vi "DiffDrivePoseEst_FillStateVector.vi"(9 "RightDist":dbl, 10 "LeftDist":dbl, 11 "InitialPose":T2={"TRANSLATION"={"X"=0.0, "Y"=0.0}, "ROTATION"={"VALUE"=0.0, "COS"=1.0, "SIN"=0.0}} {"ROTATION"."SIN" format="%13.4f"; "ROTATION"."COS" format="%13.4f"; "ROTATION"."VALUE" format="%13.4f"; "TRANSLATION"."Y" format="%14.3f"; "TRANSLATION"."X" format="%14.3f"}) -> (3 "output matrix":T1)   [LabVIEW 2019, in "Trajectory_Library.lvlib"]
doc: "Create a vector with the current robot pose, encoder distances, and gyro\n\nInputs:\n - initialPose -- robot pose\n - LeftDist -- left encoder distance\n - RightDist -- right encoder distance\n\nOutputs:\n - output Matrix -- filled matrix."
uses:
  Trajectory_Library.lvlib
  POSE2D.ctl
  TRANSLATION2D.ctl
  ROTATION2D.ctl
  <vilib>/Analysis/Matrix/Datatypes/RealMatrix.ctl
  MatBuilder_Create.vi
  <vilib>/Analysis/Matrix/NI_Matrix.lvlib
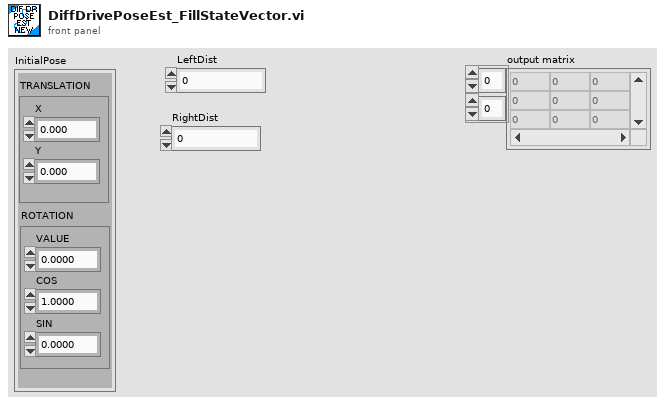
[diagram p1: front panel]
types:
  T1 = typedef "NI_Matrix.lvlib/RealMatrix.ctl" = dbl[][]
  T2 = typedef "Trajectory_Library.lvlib/POSE2D.ctl" = cluster{"TRANSLATION":T3, "ROTATION":T4}
  T3 = typedef "Trajectory_Library.lvlib/TRANSLATION2D.ctl" = cluster{"X":dbl, "Y":dbl}
  T4 = typedef "Trajectory_Library.lvlib/ROTATION2D.ctl" = cluster{"VALUE":dbl, "COS":dbl, "SIN":dbl}
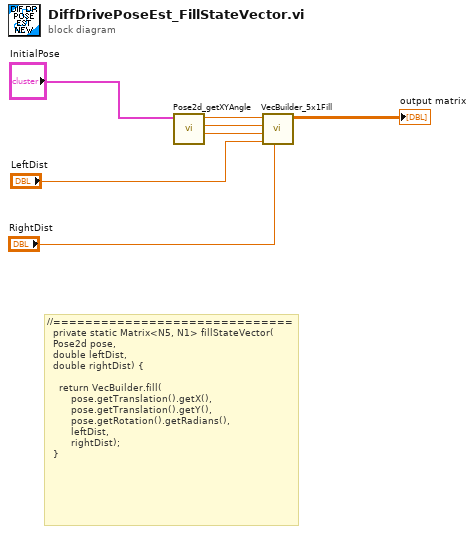
[diagram p0: block diagram]
diagram:
  # "//==============================\n  private static Matrix<N5, N1> fillStateVector(\n\t\tPose2d pose, \n\t\tdouble leftDist, \n\t\tdouble rightDist) {\n\n    return VecBuilder.fill(\n        pose.getTranslation().getX(),\n        pose.getTranslation().getY(),\n        pose.getRotation().getRadians(),\n        leftDist,\n        rightDist);\n  }"
  n1 = call "Pose2d_getXYAngle.vi"("in POSE"="InitialPose") -> ("Angle"=w4:dbl, "Y"=w5:dbl, "X"=w6:dbl)  [unwired: 8 in]
  n2 = call "VecBuilder_5x1Fill.vi"("R4"="RightDist", "R3"="LeftDist", "R2"=w4, "R1"=w5, "R0"=w6) -> ("output matrix"=→"output matrix":T1)  [unwired: 6 in]
